vi "Cleanup.vi"(8 "error in (no error)":errorcluster, 11 "Panel in":refnum<class "Panel.lvclass">) -> (0 "error out":errorcluster)   [LabVIEW 2020, in "OOPanel.lvlib" / "Panel.lvclass"]
uses:
  Panel.lvclass
  Panel.lvclass/Panel.ctl
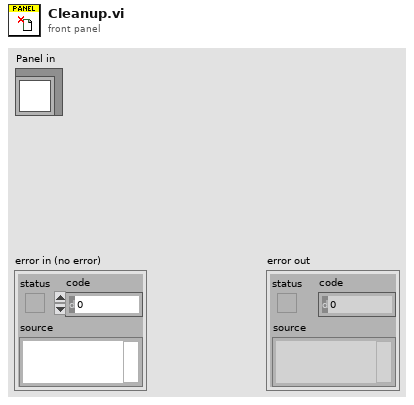
[diagram p1: front panel]
types:
  T1 = typedef "OOPanel.lvlib/Panel.lvclass/Ref Data.ctl" = cluster{"Panel Events":T2, "Panel Ref":refnum<vi>, "SubPanel":refnum<vi>, "Close":bool, "Running":bool, "State":T3}
  T2 = typedef "OOPanel.lvlib/Panel.lvclass/Panel Events.ctl" = cluster{"Visbility":refnum<user-event>, "Close":refnum<user-event>}
  T3 = typedef "OOPanel.lvlib/Panel.lvclass/Visibility State.ctl" = enum16{"Idle", "Closed", "Hidden", "Visible", "Subpanel"}
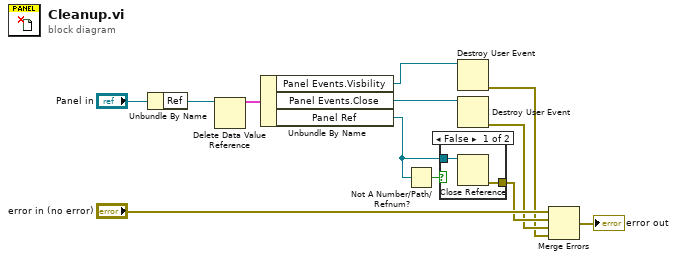
[diagram p0: block diagram]
diagram:
  n1 = Unbundle By Name("Panel in") -> ("Ref"=w11:refnum<data-value>)
  n2 = Delete Data Value Reference(data value reference=w11) -> (data value=w10:T1)  [unwired: 1 in, 1 out]
  n3 = Unbundle By Name(w10) -> ("Panel Events.Visbility"=w6:refnum<user-event>, "Panel Events.Close"=w7:refnum<user-event>, "Panel Ref"=w9:refnum<vi>)
  n4 = Not A Number/Path/Refnum?(number/path/refnum=w9) -> (NaN/Path/Refnum?=w8:bool)
  n5 = case shown="False" w8 {
    tunnel: w9 -> [w14 _]
    tunnel: [w13 _] -> w4
    frame False {
      n6 = Close Reference(reference=w14) -> (error out=w13:errorcluster)  [unwired: 1 in]
    }
    frame True {
    }
  }
  n7 = Destroy User Event(user event=w6) -> (error out=w2:errorcluster)  [unwired: 1 in]
  n8 = Destroy User Event(user event=w7) -> (error out=w3:errorcluster)  [unwired: 1 in]
  n9 = Merge Errors("error in (no error)", w4, w3, w2) -> (→"error out":errorcluster)
